vi "User Access Level FGV - Copy.vi"(7 "User Level Cmd":T1, 8 "Error In":errorcluster, 10 "User Name":string) -> (0 "Error Out":errorcluster, 1 "User Level":string)   [LabVIEW 2018]
doc: "This FGV holds the Access Level for the user currently logged in. It executes the following methods:\n\n1. <B>Read User Access Level File:</B> Reads a tab-delimited text file containing User Names and corresponding Access Levels.\n2. <B>Set Current Access Level:</B> Sets the Access level for the User Name input.\n3. <B>Get Current Access Level:</B> Returns the Access level for the current User."
uses:
  User Level Cmd.ctl
  <vilib>/Utility/file.llb/Read From Spreadsheet File (string).vi
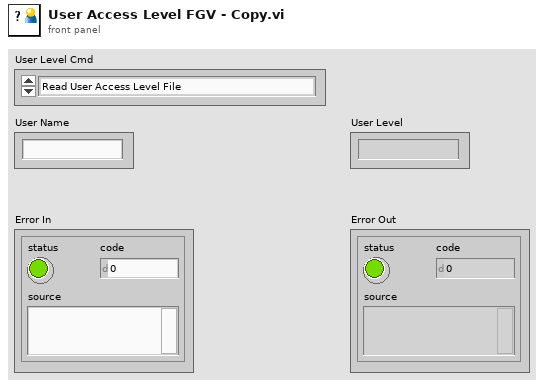
[diagram p1: front panel]
types:
  T1 = typedef "User Level Cmd.ctl" = enum16{"Read User Access Level File", "Set Current User", "Get User Access Level"}
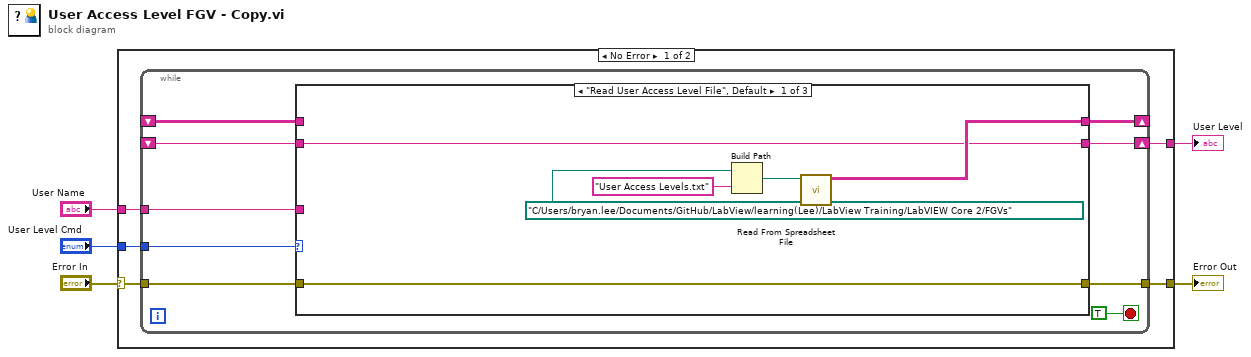
[diagram p0: block diagram]
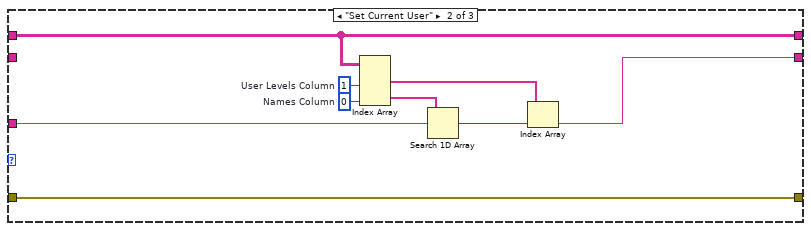
[diagram p2: hidden frame]
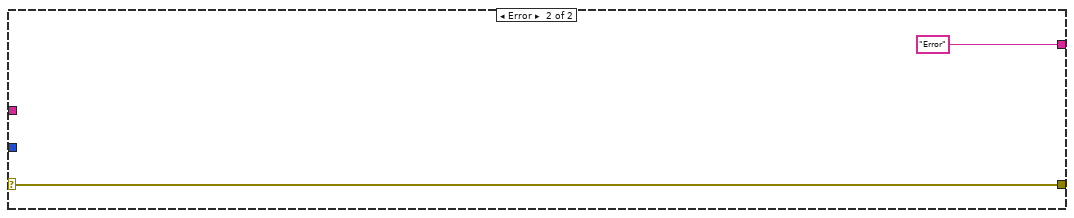
[diagram p4: hidden frame]
diagram:
  n1 = case shown="No Error" "Error In" {
    selector: "Error In" -> [w6 w39]
    tunnel: "User Level Cmd" -> [w10 _]
    tunnel: [w9 w39] -> w4
    tunnel: "User Name" -> [w8 _]
    tunnel: [w7 "Error" ("String")] -> w2
    frame No Error {
      n2 = while {
        tunnel: w10 -> [w18]
        tunnel: [w17] -> w9
        tunnel: w6 -> [w16]
        shift-right: [w15] -> _
        shift-left: _ -> [w14]
        tunnel: w8 -> [w13]
        shift-right: [w12] -> w7
        shift-left: _ -> [w11]
        stop <- TRUE stop-if-true
        n3 = case shown="\"Read User Access Level File\", Default" w18 {
          tunnel: [w25 w34 w37] -> w17
          tunnel: w16 -> [w25 w34 w37]
          tunnel: [w22 w33 w36] -> w15
          tunnel: w14 -> [_ w33 w36]
          tunnel: w13 -> [_ w31 _]
          tunnel: [w21 w27 w35] -> w12
          tunnel: w11 -> [w21 _ w35]
          frame "Read User Access Level File", Default {
            n4 = Build Path(base path=path "C:/Users/bryan.lee/Documents/GitHub/LabView/learning(Lee)/LabView Training/LabVIEW Core 2/FGVs", name or relative path="User Access Levels.txt") -> (appended path=w23:path)
            n5 = call-poly <vilib>:"Read From Spreadsheet File.vi"("file path (dialog if empty)"=w23) -> ("all rows"=w22:string[][])  [unwired: 6 in, 4 out]
          }
          frame "Set Current User" {
            w30 = 1  # User Levels Column
            w32 = 0  # Names Column
            n6 = Index Array "Index Array"(array=w33, index (col) #1=w30, index (col) #2=w32) -> (element #1=w28:string[], element #2=w26:string[])  [unwired: 2 in]
            n7 = Search 1D Array(1D array=w26, element=w31) -> (index of element=w29:i32)  [unwired: 1 in]
            n8 = Index Array "Index Array"(array=w28, index=w29) -> (element=w27:string)
          }
          frame "Get User Access Level" {
          }
        }
      }
    }
    frame Error {
    }
  }
  "User Level" <- w2
  "Error Out" <- w4
